vi "HEWH Trim FHD Data.vi"(8 "error in (no error)":errorcluster, 10 "Decrement Amount":i32, 11 "Remove 15 Seconds Input in":T1 {"Hot Water Total (Gal)" format="%#.6f"; "Software Elapsed Time (s)" format="%#.6f"; "Cold Water Total (Gal)" format="%#.6f"}) -> (0 "error out":errorcluster, 3 "Remove 15 Seconds Input out":T1 {"Hot Water Total (Gal)" format="%#.6f"; "Software Elapsed Time (s)" format="%#.6f"; "Cold Water Total (Gal)" format="%#.6f"})   [LabVIEW 2023]
uses:
  Type Definitions/HEWH Remove 15 Seconds.ctl
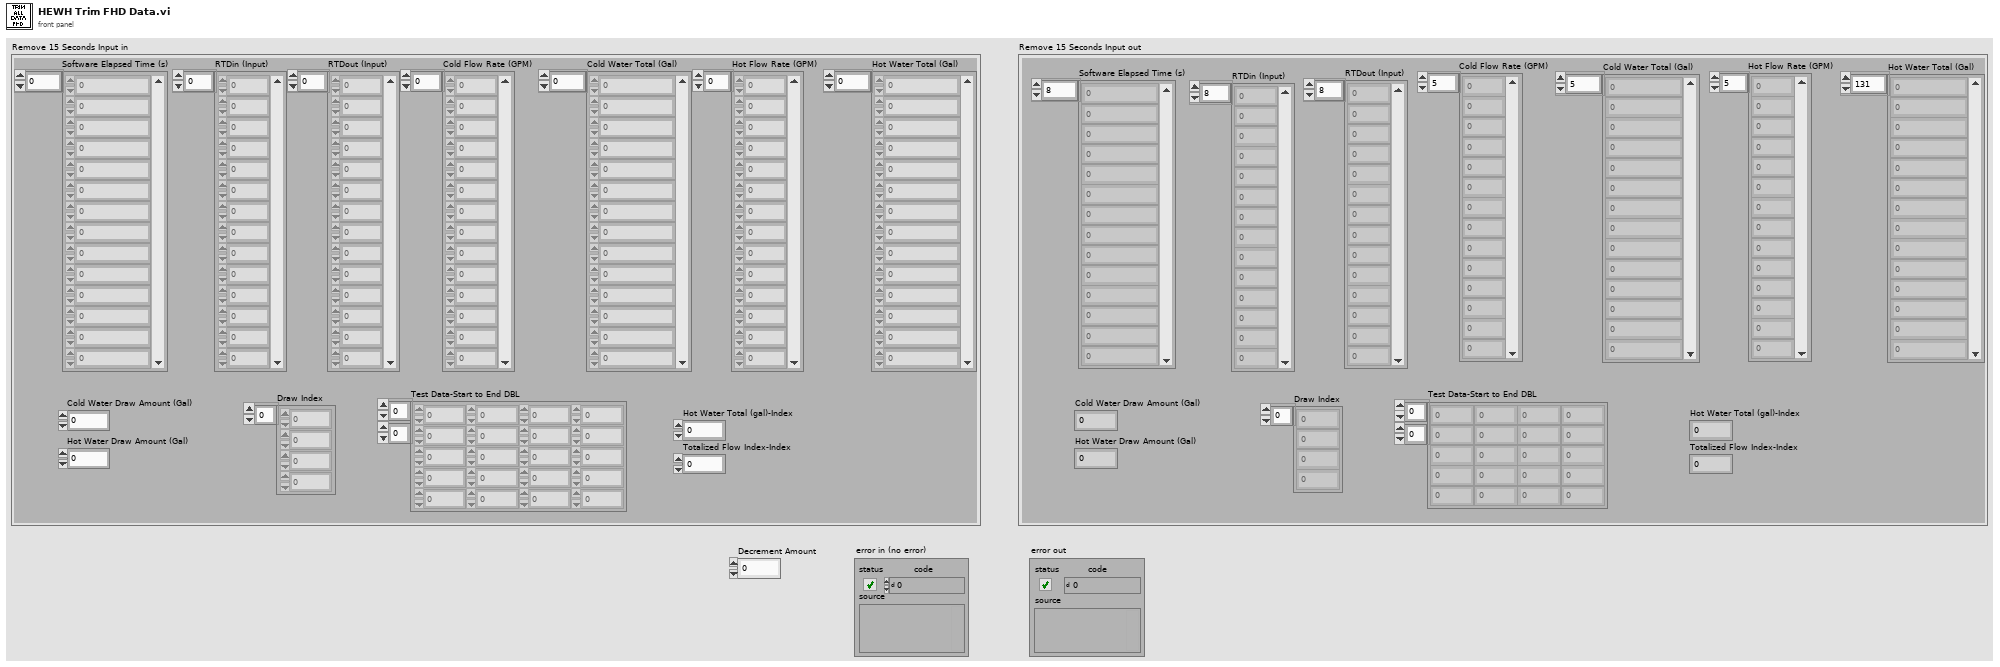
[diagram p1: front panel]
types:
  T1 = typedef "HEWH Remove 15 Seconds.ctl" = cluster{"Cold Water Total (Gal)":dbl[], "Software Elapsed Time (s)":dbl[], "RTDin (Input)":dbl[], "RTDout (Input)":dbl[], "Cold Flow Rate (GPM)":dbl[], "Hot Flow Rate (GPM)":dbl[], "Hot Water Total (Gal)":dbl[], "Cold Water Draw Amount (Gal)":dbl, "Hot Water Draw Amount (Gal)":dbl, "Draw Index":i32[], "Test Data-Start to End DBL":dbl[][], "Hot Water Total (gal)-Index":i32, "Totalized Flow Index-Index":i32}
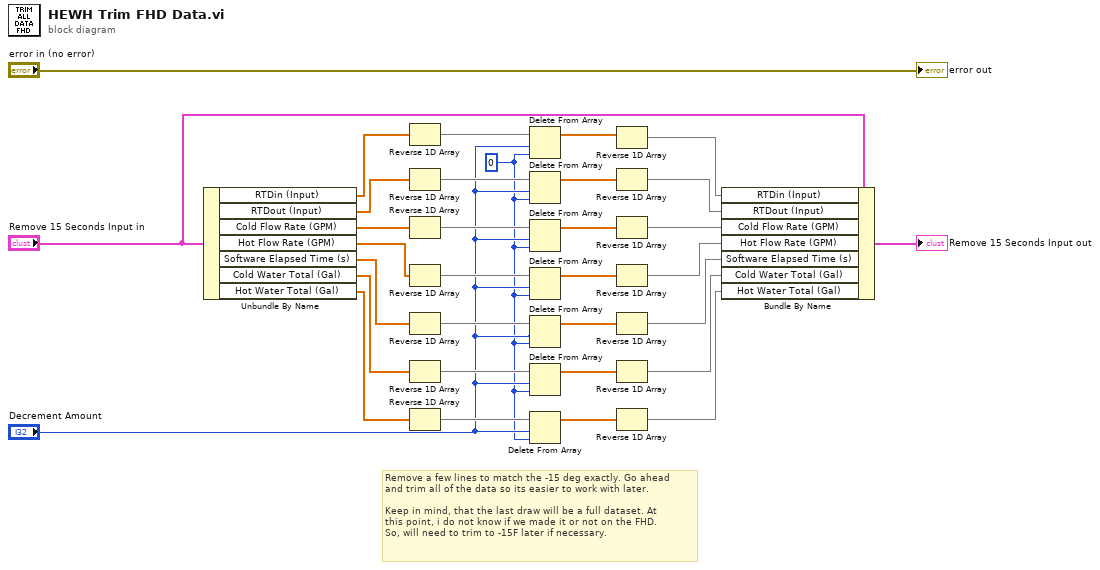
[diagram p0: block diagram]
diagram:
  w1 = 0 ("index")
  # "Remove a few lines to match the -15 deg exactly. Go ahead\nand trim all of the data so its easier to work with later.\n\nKeep in mind, that the last draw will be a full dataset. At \nthis point, i do not know if we made it or not on the FHD. \nSo, will need to trim to -15F later if necessary."
  n1 = Unbundle By Name("Remove 15 Seconds Input in") -> ("RTDin (Input)"=w23:dbl[], "RTDout (Input)"=w22:dbl[], "Cold Flow Rate (GPM)"=w21:dbl[], "Hot Flow Rate (GPM)"=w20:dbl[], "Software Elapsed Time (s)"=w19:dbl[], "Cold Water Total (Gal)"=w18:dbl[], "Hot Water Total (Gal)"=w17:dbl[])
  n2 = Reverse 1D Array(array=w23) -> (reversed array=w30:dbl[])
  n3 = Reverse 1D Array(array=w22) -> (reversed array=w29:dbl[])
  n4 = Reverse 1D Array(array=w21) -> (reversed array=w28:dbl[])
  n5 = Reverse 1D Array(array=w20) -> (reversed array=w27:dbl[])
  n6 = Reverse 1D Array(array=w19) -> (reversed array=w26:dbl[])
  n7 = Reverse 1D Array(array=w18) -> (reversed array=w25:dbl[])
  n8 = Reverse 1D Array(array=w17) -> (reversed array=w24:dbl[])
  n9 = Delete From Array(array=w30, length="Decrement Amount", index=w1) -> (array with subset deleted=w16:dbl[])  [unwired: 1 out]
  n10 = Delete From Array(array=w29, length="Decrement Amount", index=w1) -> (array with subset deleted=w15:dbl[])  [unwired: 1 out]
  n11 = Delete From Array(array=w28, length="Decrement Amount", index=w1) -> (array with subset deleted=w14:dbl[])  [unwired: 1 out]
  n12 = Delete From Array(array=w27, length="Decrement Amount", index=w1) -> (array with subset deleted=w13:dbl[])  [unwired: 1 out]
  n13 = Delete From Array(array=w26, length="Decrement Amount", index=w1) -> (array with subset deleted=w12:dbl[])  [unwired: 1 out]
  n14 = Delete From Array(array=w25, length="Decrement Amount", index=w1) -> (array with subset deleted=w11:dbl[])  [unwired: 1 out]
  n15 = Delete From Array(array=w24, length="Decrement Amount", index=w1) -> (array with subset deleted=w10:dbl[])  [unwired: 1 out]
  n16 = Reverse 1D Array(array=w16) -> (reversed array=w9:dbl[])
  n17 = Reverse 1D Array(array=w15) -> (reversed array=w8:dbl[])
  n18 = Reverse 1D Array(array=w14) -> (reversed array=w7:dbl[])
  n19 = Reverse 1D Array(array=w13) -> (reversed array=w6:dbl[])
  n20 = Reverse 1D Array(array=w12) -> (reversed array=w5:dbl[])
  n21 = Reverse 1D Array(array=w11) -> (reversed array=w4:dbl[])
  n22 = Reverse 1D Array(array=w10) -> (reversed array=w3:dbl[])
  n23 = Bundle By Name(cluster="Remove 15 Seconds Input in", "RTDin (Input)"=w9, "RTDout (Input)"=w8, "Cold Flow Rate (GPM)"=w7, "Hot Flow Rate (GPM)"=w6, "Software Elapsed Time (s)"=w5, "Cold Water Total (Gal)"=w4, "Hot Water Total (Gal)"=w3) -> (→"Remove 15 Seconds Input out":T1)
  "error out" <- "error in (no error)"
